vi "16-ParseOperator.vi"(11 "BITS in":bool[](array[boolean])) -> (2 "Packets":T1(array[cluster]), 3 "BITS out":bool[](array[boolean]))   [LabVIEW 2019, in "16.lvlib"]
uses:
  16.lvlib
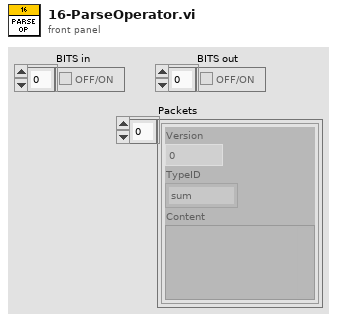
[diagram p1: front panel]
types:
  T1 = cluster{"Version":u32, "TypeID":enum16{"sum", "product", "minimum", "maximum", "literal", "greater than", "less than", "equal to"}, "Content":variant}[]
  T2 = enum8{"Total Length (bits)", "Number of Subpackets"}
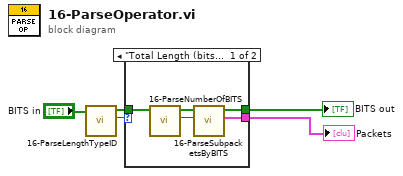
[diagram p0: block diagram]
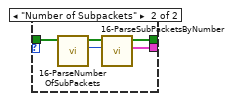
[diagram p2: hidden frame]
diagram:
  n1 = call "16-ParseLengthTypeID.vi"("BITS in in"="BITS in") -> ("Length Type ID"=w4:T2, "BITS out"=w3:bool[])  [unwired: 9 in]
  n2 = case shown="\"Total Length (bits)\"" w4 {
    tunnel: w3 -> [w7 w13]
    tunnel: [w9 w15] -> w2
    tunnel: [w10 w14] -> w1
    frame "Total Length (bits)" {
      n3 = call "16-ParseNumberOfBITS.vi"("BITS in"=w7) -> ("Number of BITS"=w6:u32, "BITS out"=w8:bool[])  [unwired: 9 in]
      n4 = call "16-ParseSubpacketsByBITS.vi"("Number of BITS"=w6, "BITS in"=w8) -> ("Sub Packets"=w10:T1, "BITS out"=w9:bool[])  [unwired: 8 in]
    }
    frame "Number of Subpackets" {
      n5 = call "16-ParseNumberOfSubPackets.vi"("BITS in"=w13) -> ("Number of Sub Packets"=w11:u32, "BITS out"=w12:bool[])  [unwired: 9 in]
      n6 = call "16-ParseSubPacketsByNumber.vi"("Number of Sub Packets"=w11, "BITS in"=w12) -> ("Sub Packets"=w14:T1, "BITS out"=w15:bool[])  [unwired: 8 in]
    }
  }
  "BITS out" <- w2
  "Packets" <- w1
